vi "AuMT8852B Block Read.vi"(8 "error in (no error)":errorcluster, 11 "VISA Session":refnum<visa-resource-name>) -> (0 "error out":errorcluster, 3 "VISA Session out":refnum<visa-resource-name>, 4 "Response":string)   [LabVIEW 2017]
doc: "Anritsu MT8852B Bluetooth Tester\n\nReads a response from the instrument in Arbitrary Block format:\n#<width of byte count><byte count><data>.\n\nOUTPUTS\nResponse - contents of the block data."
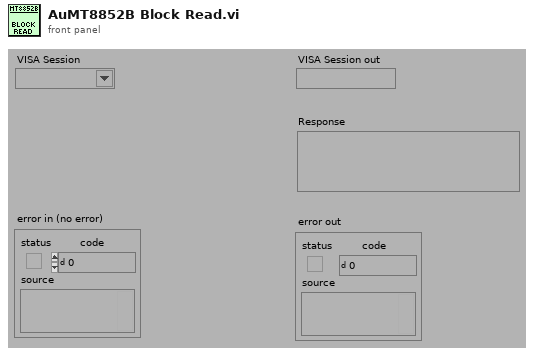
[diagram p1: front panel]
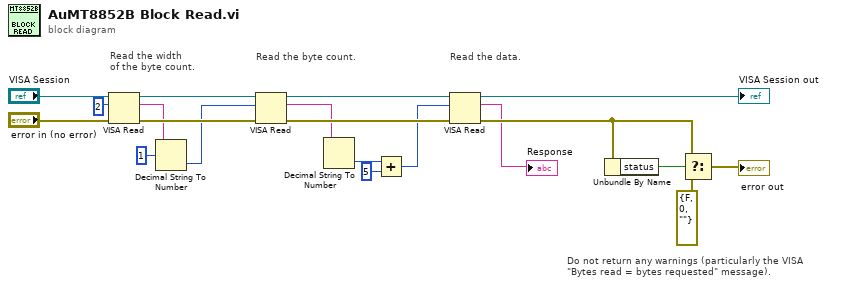
[diagram p0: block diagram]
diagram:
  # "Read the data."
  # "Read the byte count."
  # "Read the width\nof the byte count."
  # "Do not return any warnings (particularly the VISA\n\"Bytes read = bytes requested\" message)."
  n1 = VISA Read(VISA resource name="VISA Session", byte count=u32 2 ("byte count (0)"), error in (no error)="error in (no error)") -> (VISA resource name out=w13:refnum<visa-resource-name>, read buffer=w8:string, error out=w12:errorcluster)  [unwired: 1 out]
  n2 = Decimal String To Number(string=w8, offset=1) -> (number=w6:i32)  [unwired: 1 in, 1 out]
  n3 = VISA Read(VISA resource name=w13, byte count=w6, error in (no error)=w12) -> (VISA resource name out=w10:refnum<visa-resource-name>, read buffer=w5:string, error out=w11:errorcluster)  [unwired: 1 out]
  n4 = Decimal String To Number(string=w5) -> (number=w4:i32)  [unwired: 2 in, 1 out]
  n5 = Add(x=w4, y=5) -> (x+y=w3:i32)
  n6 = VISA Read(VISA resource name=w10, byte count=w3, error in (no error)=w11) -> (VISA resource name out=→"VISA Session out":refnum<visa-resource-name>, read buffer=→"Response":string, error out=w17:errorcluster)  [unwired: 1 out]
  n7 = Unbundle By Name(w17) -> ("status"=w18:bool)
  n8 = Select(t=w17, s=w18, f=errorcluster {"status"=FALSE, "code"=0, "source"=""}) -> (s? t:f=→"error out":errorcluster)
